vi "L02.vi"() -> ()   [LabVIEW 2012]
panel:
  in  "n":i32
  out "sum":i32
  out "Array":i32[](array[numeric])
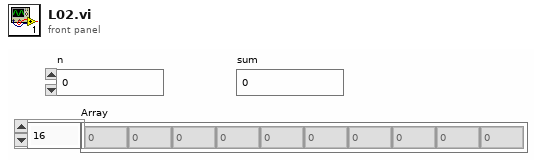
[diagram p1: front panel]
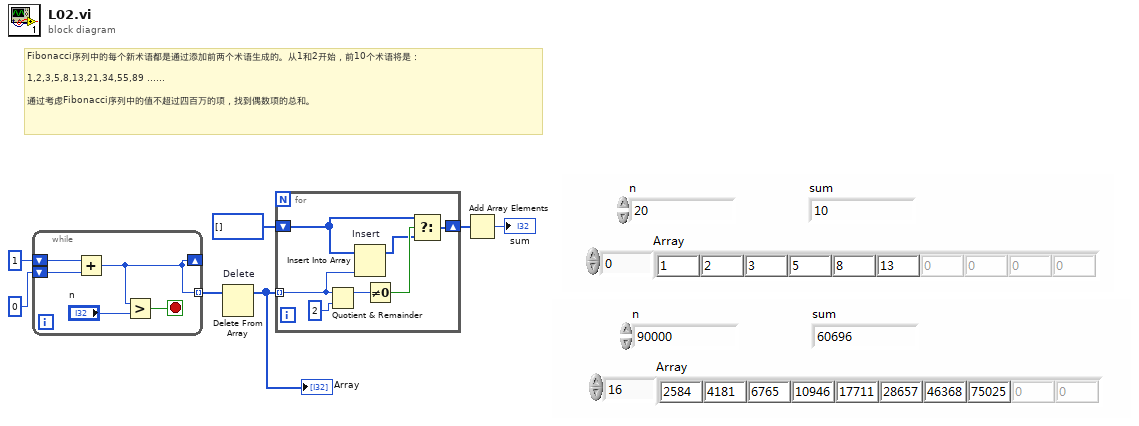
[diagram p0: block diagram]
diagram:
  # "Fibonacci序列中的每个新术语都是通过添加前两个术语生成的。从1和2开始，前10个术语将是：\n\n1,2,3,5,8,13,21,34,55,89 ......\n\n通过考虑Fibonacci序列中的值不超过四百万的项，找到偶数项的总和。"
  n1 = while {
    shift-right: [w9] -> _
    shift-left: 1 -> [w12]
    shift-left: 0 -> [w11]
    tunnel: [w9] -> w2 mode=indexing
    stop <- w10 stop-if-true
    n2 = Add(x=w12, y=w11) -> (x+y=w9:i32)
    n3 = Greater?(x=w9, y="n") -> (0:w10:bool)
  }
  n4 = Delete From Array "Delete"(array=w2) -> (array with subset deleted=w1:i32[])  [unwired: 2 in, 1 out]
  "Array" <- w1
  n5 = for {
    tunnel: w1 -> [w14] mode=indexing
    shift-right: [w13] -> w3
    shift-left: i32[] [] -> [w16]
    n6 = Quotient & Remainder(x=w14, y=2) -> (x-y*floor(x/y)=w18:i32)  [unwired: 1 out]
    n7 = Insert Into Array "Insert"(array=w16, new element=w14) -> (w15:i32[])  [unwired: 1 in]
    n8 = Not Equal To 0?(x=w18) -> (x != 0?=w17:bool)
    n9 = Select(t=w16, s=w17, f=w15) -> (s? t:f=w13:i32[])
  }
  n10 = Add Array Elements(numeric array=w3) -> (sum=→"sum":i32)
